vi "Initialize Attributes.vi"(8 "error in (no error)":errorcluster, 10 "Attribute Data":variant, 11 "CS++DMM in":refnum<class "CS++DMM.lvclass">) -> (0 "error out":errorcluster, 2 "Found?":bool, 3 "CS++DMM out":refnum<class "CS++DMM.lvclass">)   [LabVIEW 2013, in "CS++DMM.lvlib" / "CS++DMM.lvclass"]
doc: "Initialize object attribute.\n\nUnique resources should be allocated elsewhere!"
uses:
  CS++DMM.lvclass
  Core/Actors/CS++DeviceActor/CS++DeviceActor.lvclass
  Core/Actors/CS++BaseActor/CS++BaseActor.lvclass/CS++BaseActor.ctl
  Core/Classes/CS++BaseClasses/Factory/CS++Factory.lvclass
  CS++DMM.lvclass/CS++DMM.ctl
  Core/Actors/CS++BaseActor/CS++BaseActor.lvclass
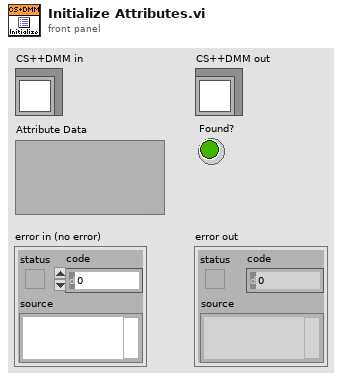
[diagram p1: front panel]
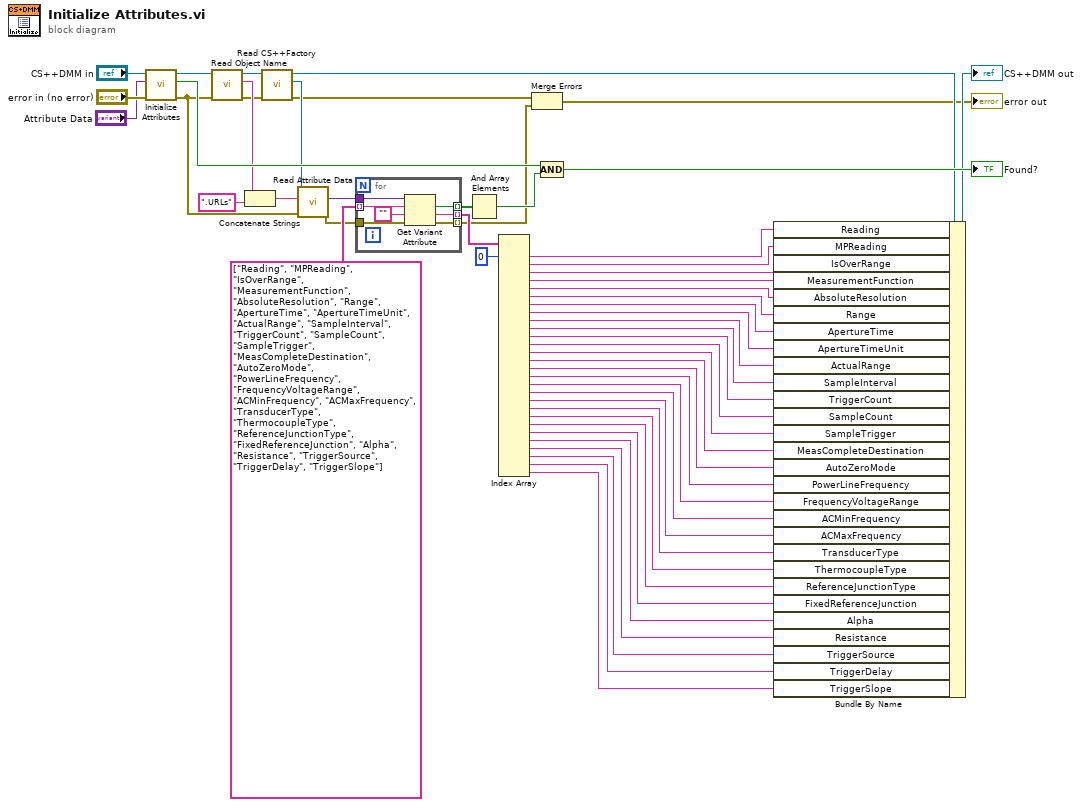
[diagram p0: block diagram]
diagram:
  n1 = call-parent "Initialize Attributes.vi"("error in (no error)"="error in (no error)", "Attribute Data"="Attribute Data", "CS++DeviceActor in"="CS++DMM in") -> ("error out"=w35:errorcluster, "Found?"=w50:bool, "CS++DeviceActor out"=w46:refnum<class "CS++DMM.lvclass">)  [unwired: 6 in]
  n2 = call "Read Object Name.vi"("error in (no error)"=w35, "CS++BaseActor in"=w46) -> ("error out"=w39:errorcluster, "Object Name"=w45:string, "CS++BaseActor out"=w47:refnum<class "CS++DMM.lvclass">)  [unwired: 7 in]
  n3 = Concatenate Strings(w45, ".URLs" ("string")) -> (w48:string)
  n4 = call "Read CS++Factory.vi"("error in (no error)"=w39, "CS++BaseActor in"=w47) -> ("error out"=w38:errorcluster, "CS++Factory"=w44:refnum<class "CS++Factory.lvclass">, "CS++BaseActor out"=w42:refnum<class "CS++DMM.lvclass">)  [unwired: 7 in]
  n5 = call-dynamic "Read Attribute Data.vi"("error in (no error)"=w35, "Object Name"=w48, "CS++Factory in"=w44) -> ("error out"=w34:errorcluster, "Attribute Data"=w37:variant)  [unwired: 6 in, 1 out]
  n6 = for {
    tunnel: w37 -> [w59]
    tunnel: string[] ["Reading", "MPReading", "IsOverRange", "MeasurementFunction", "AbsoluteResolution", "Range", "ApertureTime", "ApertureTimeUnit", "ActualRange", "SampleInterval", "TriggerCount", "SampleCount", "SampleTrigger", "MeasCompleteDestination", "AutoZeroMode", "PowerLineFrequency", "FrequencyVoltageRange", "ACMinFrequency", "ACMaxFrequency", "TransducerType", "ThermocoupleType", "ReferenceJunctionType", "FixedReferenceJunction", "Alpha", "Resistance", "TriggerSource", "TriggerDelay", "TriggerSlope"] -> [w58] mode=indexing
    tunnel: w34 -> [w57]
    tunnel: [w56] -> w26 mode=indexing
    tunnel: [w55] -> w33 mode=indexing
    tunnel: [w54] -> w31 mode=indexing
    n7 = Get Variant Attribute(Variant=w59, name=w58, default value (empty Variant)="", error in=w57) -> (found=w55:bool, value=w54:string, error out=w56:errorcluster)  [unwired: 1 out]
  }
  n8 = And Array Elements(Boolean array=w33) -> (logical AND=w32:bool)
  n9 = Index Array(array=w31, index #1=0 ("index")) -> (element #1=w29:string, element #2=w28:string, element #3=w27:string, element #4=w25:string, element #5=w24:string, element #6=w23:string, element #7=w22:string, element #8=w21:string, element #9=w20:string, element #10=w19:string, element #11=w18:string, element #12=w17:string, element #13=w16:string, element #14=w15:string, element #15=w14:string, element #16=w13:string, element #17=w12:string, element #18=w11:string, element #19=w10:string, element #20=w9:string, element #21=w8:string, element #22=w7:string, element #23=w6:string, element #24=w5:string, element #25=w4:string, element #26=w3:string, element #27=w2:string, element #28=w1:string)  [unwired: 27 in]
  n10 = Merge Errors(w38, w26) -> (→"error out":errorcluster)
  n11 = Compound Arithmetic op=AND(w50, w32) -> (→"Found?":bool)
  n12 = Bundle By Name(cluster=w42, "Reading"=w29, "MPReading"=w28, "IsOverRange"=w27, "MeasurementFunction"=w25, "AbsoluteResolution"=w24, "Range"=w23, "ApertureTime"=w22, "ApertureTimeUnit"=w21, "ActualRange"=w20, "SampleInterval"=w19, "TriggerCount"=w18, "SampleCount"=w17, "SampleTrigger"=w16, "MeasCompleteDestination"=w15, "AutoZeroMode"=w14, "PowerLineFrequency"=w13, "FrequencyVoltageRange"=w12, "ACMinFrequency"=w11, "ACMaxFrequency"=w10, "TransducerType"=w9, "ThermocoupleType"=w8, "ReferenceJunctionType"=w7, "FixedReferenceJunction"=w6, "Alpha"=w5, "Resistance"=w4, "TriggerSource"=w3, "TriggerDelay"=w2, "TriggerSlope"=w1) -> (→"CS++DMM out":refnum<class "CS++DMM.lvclass">)
